vi "DI Command Mode Select.vi"(8 "Configuration":T1, 11 "InjCommand in":T2[](array[typedef]) {"EPT Precharge Profile Index" max=15; "EPT Precharge Duration [s]" min=0 format="%#_4p"; "Default Profile Index" max=15; "Cal Increment [s]" format="%#_3p"; "TMP Command Sequence"."Profile Index" max=7; "TMP Command Sequence"."Duration [s]" min=0 max=100 format="%#_3p"; "Cal Pulses" max=511; "EPT Skip Index" max=7; "EPT Angles"."Profile Index" max=7; "EPT Angles"."Duration [s]" min=0 max=100 format="%#_3p"; "Cal Duration [s]" format="%#_3p"; "Cal Freq [Hz]" format="%#_3p"}) -> (0 "Pump Enabled":bool, 1 "N Injectors":i32, 3 "InjCommand out":T2[](array[typedef]) {"EPT Precharge Profile Index" max=15; "EPT Precharge Duration [s]" min=0 format="%#_4p"; "Default Profile Index" max=15; "Cal Increment [s]" format="%#_3p"; "TMP Command Sequence"."Profile Index" max=7; "TMP Command Sequence"."Duration [s]" min=0 max=100 format="%#_3p"; "Cal Pulses" max=511; "EPT Skip Index" max=7; "EPT Angles"."Profile Index" max=7; "EPT Angles"."Duration [s]" min=0 max=100 format="%#_3p"; "Cal Duration [s]" format="%#_3p"; "Cal Freq [Hz]" format="%#_3p"})   [LabVIEW 2016, in "DCM System Explorer.lvlib"]
uses:
  DCM System Explorer.lvlib
  <vilib>/Powertrain Controls/Device Drivers/DCM/DI/RT/Command.ctl
  <vilib>/Powertrain Controls/Device Drivers/DCM/DI/FPGA/Mode.ctl
  <vilib>/Powertrain Controls/Device Drivers/DCM/Rev0/FPGA/Digital Channel.ctl
  <vilib>/Powertrain Controls/Device Drivers/DCM/DI/RT/Command Sequence.ctl
  <vilib>/Powertrain Controls/Device Drivers/DCM/DI/RT/Angle Control.ctl
  <vilib>/Powertrain Controls/Device Drivers/DCM/Rev0/FPGA/DI - Bank Configuration.ctl
  <vilib>/Powertrain Controls/Device Drivers/DCM/DI/RT/DCM - RT - DI.lvlib
  <vilib>/Powertrain Controls/Device Drivers/DCM/DI/FPGA/DCM - FPGA - DI.lvlib
  <vilib>/Powertrain Controls/Device Drivers/DCM/Rev0/FPGA/DCM - FPGA.lvlib
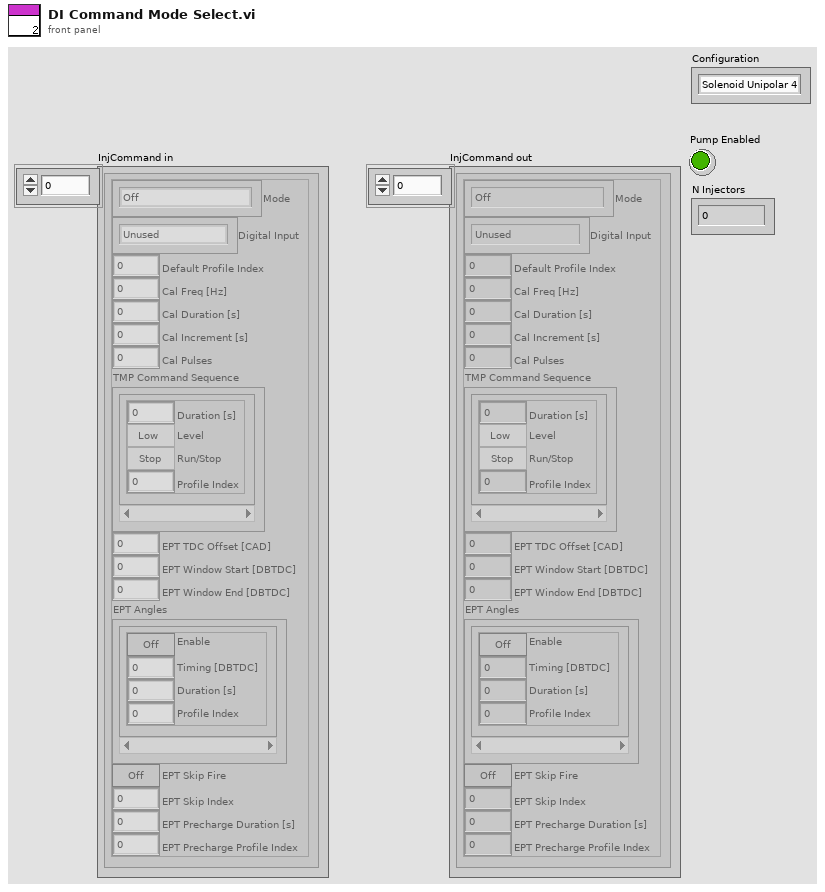
[diagram p1: front panel]
types:
  T1 = typedef "DCM - FPGA.lvlib/DI - Bank Configuration.ctl" = enum8{"Solenoid Unipolar 4", "Solenoid Unipolar 7 (Muxed)", "Solenoid Unipolar 8 (Muxed)", "Solenoid Bipolar 2", "Solenoid Bipolar 3 (Muxed)", "Piezo Unipolar 2", "Piezo Unipolar 3 (Muxed)", "Piezo Unipolar 4 (Muxed)", "Piezo Bipolar 2", "Piezo Bipolar 3 (Muxed)"}
  T2 = typedef "DCM - RT - DI.lvlib/Command.ctl" = cluster{"Mode":T3, "Digital Input":T4, "Default Profile Index":u8, "Cal Freq [Hz]":sgl, "Cal Duration [s]":sgl, "Cal Increment [s]":sgl, "Cal Pulses":u16, "TMP Command Sequence":T5[], "EPT TDC Offset [CAD]":sgl, "EPT Window Start [DBTDC]":sgl, "EPT Window End [DBTDC]":sgl, "EPT Angles":T6[], "EPT Skip Fire":bool, "EPT Skip Index":u8, "EPT Precharge Duration [s]":sgl, "EPT Precharge Profile Index":u8}
  T3 = typedef "DCM - FPGA - DI.lvlib/Mode.ctl" = enum8{"Off", "Direct", "Calibration", "Triggered Multi-Pulse", "Engine Position Tracking"}
  T4 = typedef "DCM - FPGA.lvlib/Digital Channel.ctl" = enum8{"Unused", "User OS", "Diff IO 1", "Diff IO 2", "Diff IO 3", "Diff IO 4", "Diff IO 5", "Diff IO 6", "Diff IO 7", "Diff IO 8", "Aux 1", "Aux 2", "Aux 3", "Aux 4", "Aux 5", "Aux 6", "Aux 7", "Aux 8", "Aux 9", "Aux 10", "Aux 11", "Aux 12", "Aux 13", "Aux 14", "Aux 15", "Aux 16"}
  T5 = typedef "DCM - RT - DI.lvlib/Command Sequence.ctl" = cluster{"Duration [s]":sgl, "Level":bool, "Run/Stop":bool, "Profile Index":u8}
  T6 = typedef "DCM - RT - DI.lvlib/Angle Control.ctl" = cluster{"Enable":bool, "Timing [DBTDC]":sgl, "Duration [s]":sgl, "Profile Index":u8}
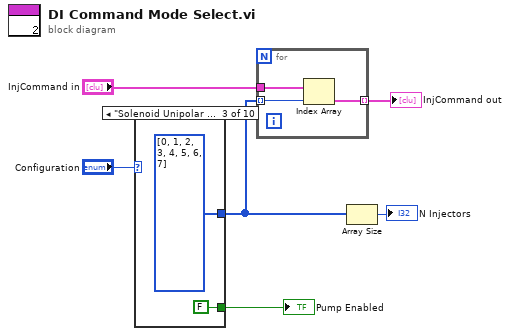
[diagram p0: block diagram]
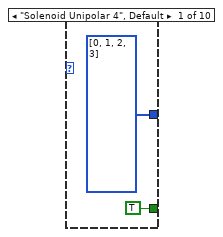
[diagram p2: hidden frame]
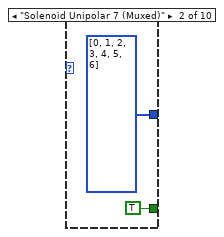
[diagram p3: hidden frame]
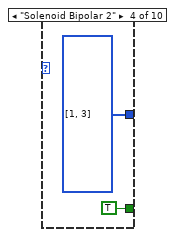
[diagram p4: hidden frame]
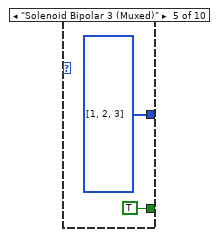
[diagram p5: hidden frame]
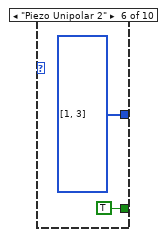
[diagram p6: hidden frame]
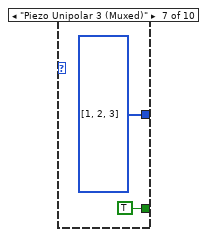
[diagram p7: hidden frame]
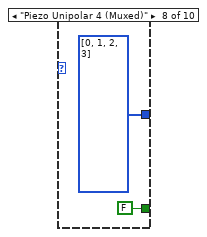
[diagram p8: hidden frame]
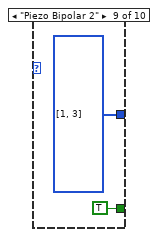
[diagram p9: hidden frame]
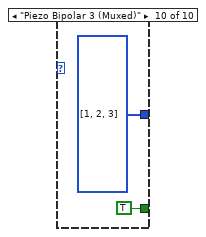
[diagram p10: hidden frame]
diagram:
  n1 = case shown="\"Solenoid Unipolar 8 (Muxed)\"" "Configuration" {
    tunnel: [i32[] [0, 1, 2, 3] i32[] [0, 1, 2, 3, 4, 5, 6] i32[] [0, 1, 2, 3, 4, 5, 6, 7] i32[] [1, 3] i32[] [1, 2, 3] i32[] [1, 3] i32[] [1, 2, 3] i32[] [0, 1, 2, 3] i32[] [1, 3] i32[] [1, 2, 3]] -> w2
    tunnel: [TRUE ("Pump Enabled") TRUE ("Pump Enabled") FALSE ("Pump Enabled") TRUE ("Pump Enabled") TRUE ("Pump Enabled") TRUE ("Pump Enabled") TRUE ("Pump Enabled") FALSE ("Pump Enabled") TRUE ("Pump Enabled") TRUE ("Pump Enabled")] -> w3
    frame "Solenoid Unipolar 4", Default {
    }
    frame "Solenoid Unipolar 7 (Muxed)" {
    }
    frame "Solenoid Unipolar 8 (Muxed)" {
    }
    frame "Solenoid Bipolar 2" {
    }
    frame "Solenoid Bipolar 3 (Muxed)" {
    }
    frame "Piezo Unipolar 2" {
    }
    frame "Piezo Unipolar 3 (Muxed)" {
    }
    frame "Piezo Unipolar 4 (Muxed)" {
    }
    frame "Piezo Bipolar 2" {
    }
    frame "Piezo Bipolar 3 (Muxed)" {
    }
  }
  "Pump Enabled" <- w3
  n2 = for {
    tunnel: "InjCommand in" -> [w29]
    tunnel: [w28] -> w4 mode=indexing
    tunnel: w2 -> [w27] mode=indexing
    n3 = Index Array(array=w29, index=w27) -> (element=w28:T2)
  }
  "InjCommand out" <- w4
  n4 = Array Size(array=w2) -> (size(s)=→"N Injectors":i32)
